vi "Result_Test.vi"(8 "error in (no error)":errorcluster caption="entrée d'erreur (pas d'erreur)", 11 "Delay en entrée":refnum<class "Operator_Control.lvclass">) -> (0 "error out":errorcluster caption="sortie d'erreur", 3 "Delay en sortie":refnum<class "Operator_Control.lvclass">)   [LabVIEW 2020, in "Library Test.lvlib" / "Operator_Control.lvclass"]
uses:
  Operator_Control.lvclass
  C:/Users/ngarcin/OneDrive - Altyor/Standard TB/Class/Test/Test (Default)/Test (Default).lvclass
  Test_Without_Instr/Test_Without_Inst.lvclass
  Operator_Control.lvclass/Operator_Control.ctl
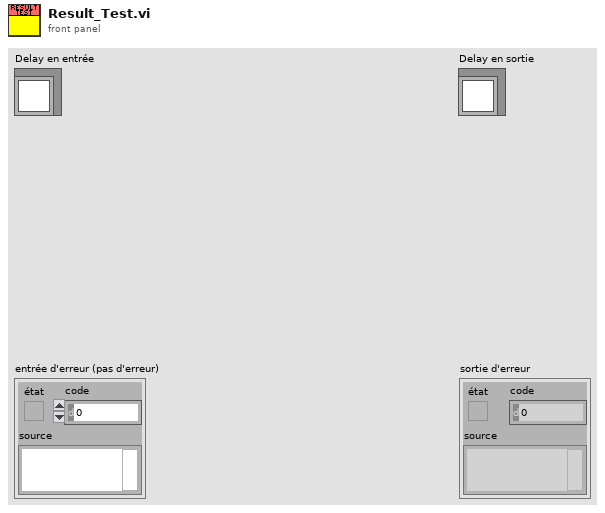
[diagram p1: front panel]
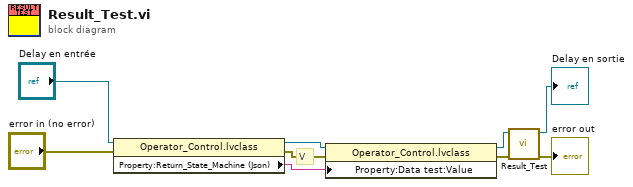
[diagram p0: block diagram]
diagram:
  # "V"
  n1 = property class="Operator_Control.lvclass"(reference="Delay en entrée", error in="error in (no error)") -> (reference out=w3:refnum<class "Operator_Control.lvclass">, error out=w5:errorcluster, "Property:Return_State_Machine (Json)"=w1:string)
  n2 = property class="Operator_Control.lvclass"(reference=w3, error in=w5, "Property:Data test:Value"=w1) -> (reference out=w2:refnum<class "Operator_Control.lvclass">, error out=w4:errorcluster)
  n3 = call-parent "Result_Test.vi"("error in (no error)"=w4, "Test_Without_Inst en entrée"=w2) -> ("error out"=→"error out":errorcluster, "Test_Without_Inst en sortie"=→"Delay en sortie":refnum<class "Operator_Control.lvclass">)  [unwired: 8 in]
